vi "add_TOP_clause_to_DELETE_statement.vi"(7 "nmb_of_top_rows (all)":i32, 8 "error_in":errorcluster, 11 "DELETE_statement_in":string) -> (0 "error_out":errorcluster, 3 "DELETE_statement_out":string)   [LabVIEW 2019]
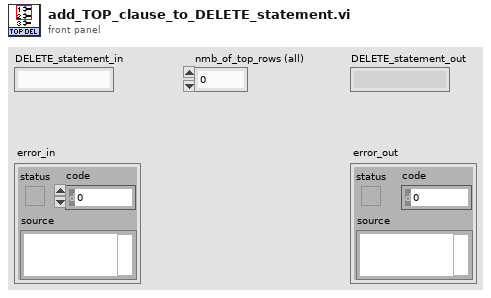
[diagram p1: front panel]
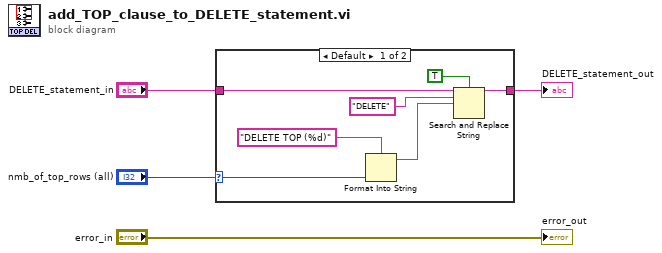
[diagram p0: block diagram]
diagram:
  n1 = case shown="Default" "nmb_of_top_rows (all)" {
    selector: "nmb_of_top_rows (all)" -> [w5 _]
    tunnel: "DELETE_statement_in" -> [w9 w12]
    tunnel: [w10 w12] -> w4
    frame Default {
      n2 = Format Into String(format string="DELETE TOP (%d)", w5) -> (resulting string=w7:string)  [unwired: 2 in, 1 out]
      n3 = Search and Replace String(case sensitive?=TRUE ("ignore case? (F)"), input string=w9, search string="DELETE", replace string=w7) -> (result string=w10:string)  [unwired: 4 in, 3 out]
    }
    frame 0 {
    }
  }
  "DELETE_statement_out" <- w4
  "error_out" <- "error_in"
